vi "Read Allow Undefinded Values.vi"(9 "Ring in":refnum<class "Ring.lvclass">) -> (3 "Ring out":refnum<class "Ring.lvclass">, 4 "Allow Undefinded Values":bool)   [LabVIEW 2014, in "Ring.lvclass"]
uses:
  Ring.lvclass
  Ring.lvclass/Ring.ctl
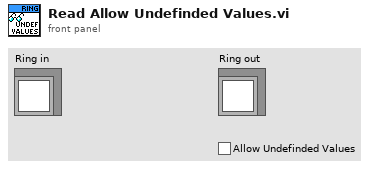
[diagram p1: front panel]
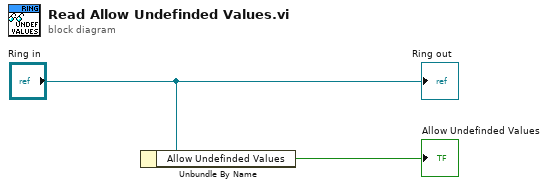
[diagram p0: block diagram]
diagram:
  n1 = Unbundle By Name("Ring in") -> ("Allow Undefinded Values"=→"Allow Undefinded Values":bool)
  "Ring out" <- "Ring in"
